vi "STM Read Message (TCP).vi"(6 "Options":T2={"Ignore Timeout Error"=TRUE, "timeout ms (1000)"=1000}, 8 "error in":errorcluster, 11 "Connection In":T4) -> (0 "error out":errorcluster, 1 "Name":T3, 2 "data string":string, 3 "Connection In":T4, 4 "Data Info":T1, 5 "Timed Out?":bool)   [LabVIEW 2015, in "J1939 Addon Shared.lvlib"]
doc: "This VI reads an incoming package of data from a host. This VI parses the package and extracts the data name and type as described in the meta data.\n\nFor the package to be parsed correctly, the meta data must be consistent in both the sender and the receiver. The data is packaged based on the existing meta data on the sender. \n\nUse the \"STM Read Meta Data\" and \"STM Write Meta Data\" VIs to ensure that both client and server have the same meta data.\n\nThe data is returned as a string. It is the responsibility of the user to cast it to the appropriate type."
uses:
  J1939 Addon Shared.lvlib
  stm_TCP Connection Info.ctl
  _SubVIs/stm_MetaDataElement.ctl
  stm_TCP Read Options.ctl
  stm_TCP Data Info.ctl
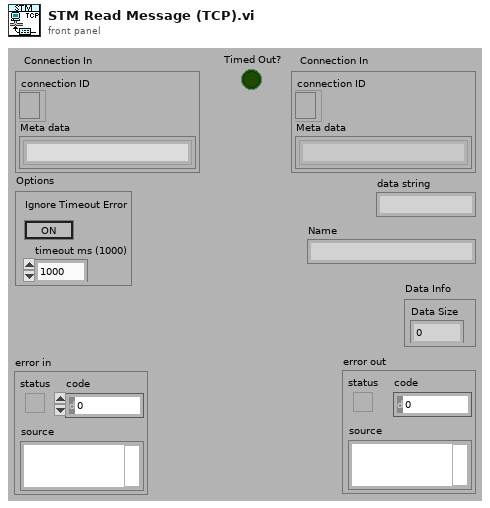
[diagram p1: front panel]
types:
  T1 = typedef "J1939 Addon Shared.lvlib/stm_TCP Data Info.ctl" = cluster{"Data Size":i32}
  T2 = typedef "J1939 Addon Shared.lvlib/stm_TCP Read Options.ctl" = cluster{"Ignore Timeout Error":bool, "timeout ms (1000)":i32}
  T3 = typedef "J1939 Addon Shared.lvlib/stm_MetaDataElement.ctl" = string
  T4 = typedef "J1939 Addon Shared.lvlib/stm_TCP Connection Info.ctl" = cluster{"connection ID":refnum<k5>, "Meta data":T3[]}
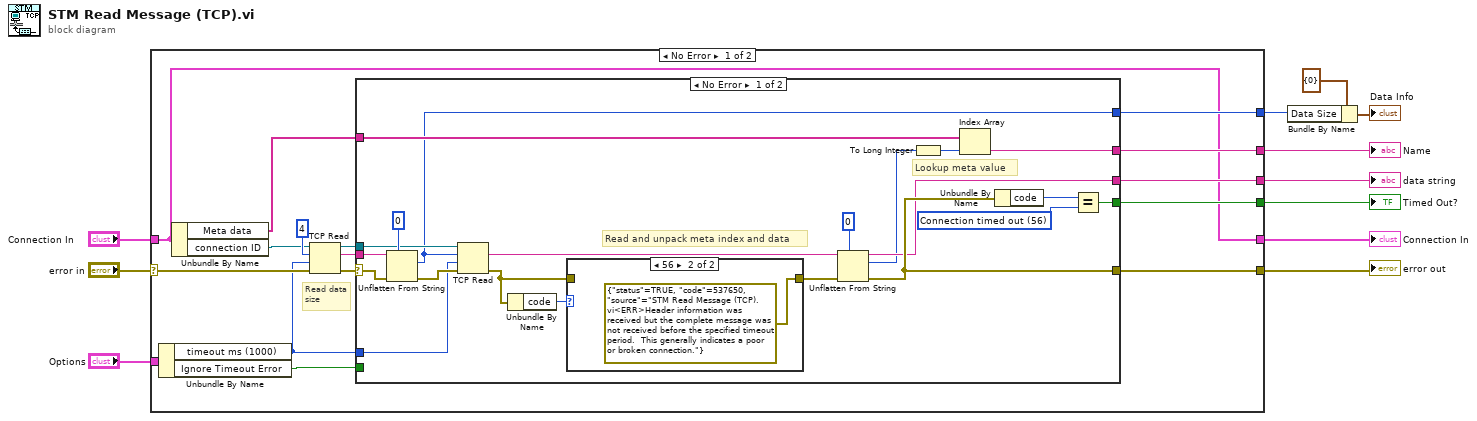
[diagram p0: block diagram]
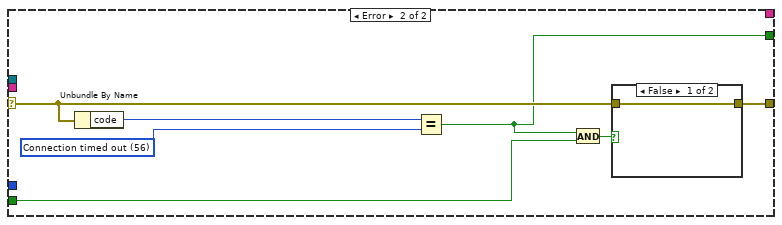
[diagram p3: hidden frame]
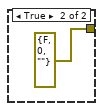
[diagram p4: hidden frame]
diagram:
  n1 = case shown="No Error" "error in" {
    selector: "error in" -> [w14 w60]
    tunnel: "Connection In" -> [w13 w61]
    tunnel: [w13 w61] -> w11
    tunnel: [w23 w60] -> w10
    tunnel: [w22 _] -> w9
    tunnel: [w21 _] -> w8
    tunnel: [w20 _] -> w7
    tunnel: [w19 _] -> w3
    tunnel: "Options" -> [w15 _]
    frame No Error {
      # "Read data size"
      n2 = Unbundle By Name(w15) -> ("timeout ms (1000)"=w12:i32, "Ignore Timeout Error"=w18:bool)
      n3 = Unbundle By Name(w13) -> ("Meta data"=w16:T3[], "connection ID"=w17:refnum<k5>)
      n4 = TCP Read(connection ID=w17, bytes to read=4, error in (no error)=w14, 9:w12) -> (connection ID out=w25:refnum<k5>, data out=w26:string, error out=w24:errorcluster)  [unwired: 1 out]
      n5 = case shown="No Error" w24 {
        selector: w24 -> [w41 w52]
        tunnel: w26 -> [w42 _]
        tunnel: w25 -> [w47 _]
        tunnel: w16 -> [w46 _]
        tunnel: [w40 w53] -> w23
        tunnel: w18 -> [_ w55]
        tunnel: [w43 w51] -> w22
        tunnel: [w39 _] -> w21
        tunnel: [w34 _] -> w20
        tunnel: [w38 _] -> w19
        tunnel: w12 -> [w28 _]
        frame No Error {
          w44 = 56 items=["No Error", "Argument Error", "Memory Full", "Out of Zone", "End of File", "File Already Open", "Generic File IO Error", "File Not Found", "File Permission Error", "Disk Full", "Duplicate Path", "Too Many Files Open", "Not Enabled", "Resource File Not Found", "Cannot Add Resource", "Resource Not Found", "Image Not Found", "Image Memory Error", "Pen Does Not Exist", "Config Bad Type", "Config Token Not Found", "Config Parse Error", "Config Memory Error", "Bad External Code Format", "Bad External Code Offset", "External Code Not Present", "Null Window", "Destroy Window Mixup", "Null Menu", "Print Aborted", "Bad Print Record", "Print Driver Error", "Windows Error During Print", "Memory Error During Print", "Print Dialog Error", "Generic Print Error", "Invalid Device Refnum", "Device Not Found", "Device Parameter Error", "Device Unit Error", "Can't Open Device", "Device Call Aborted", "Generic Error", "Cancelled By User", "Object ID Too Low", "Object ID Too High", "Object Not In Heap", "Unknown Heap", "Bad DefProc ID", "DefProc Not In Table", "Message Out Of Range", "Null Method", "Unknown Message", "Manager Call Not Supported", "Bad address", "Connection In progress", "Connection timed out", "Connection is already in progress", "Network attribute not supported", "Network error", "Address in use", "System out of memory", "Connection aborted", "Connection refused", "Connection is not connected", "Connection is already connected", "Connection closed", "Initialize error (interapplication manager)", "Bad occurrence", "Wait on unbound occurrence handler", "Occurrence queue overflow", "Bad path", "Semaphore not signaled", "Unrecognized type (interapplication manager)"] ("1st Error to Convert")
          # "Lookup meta value"
          # "Read and unpack meta index and data"
          n6 = Unflatten From String(type=0 ("bytes to read"), binary string=w42, error in (no error)=w41) -> (value=w38:i32, error out=w36:errorcluster)  [unwired: 1 in, 2 out]
          n7 = TCP Read(connection ID=w47, bytes to read=w38, error in (no error)=w36, 9:w28) -> (data out=w37:string, error out=w30:errorcluster)  [unwired: 2 out]
          n8 = Unbundle By Name(w30) -> ("code"=w29:i32)
          n9 = case shown="56" w29 {
            tunnel: w30 -> [w49 _]
            tunnel: [w49 errorcluster {"status"=TRUE, "code"=537650, "source"="STM Read Message (TCP).vi<ERR>Header information was received but the complete message was not received before the specified timeout period.  This generally indicates a poor or broken connection."} ("error out")] -> w31
            frame Default {
            }
            frame 56 {
            }
          }
          n10 = Unflatten From String(type=u16 0 ("bytes to read"), binary string=w37, error in (no error)=w31) -> (rest of the binary string=w34:string, value=w32:u16, error out=w40:errorcluster)  [unwired: 2 out]
          n11 = To Long Integer(number=w32) -> (32bit integer=w33:i32)
          n12 = Index Array(array=w46, index=w33) -> (element=w39:T3)
          n13 = Unbundle By Name(w40) -> ("code"=w45:i32)
          n14 = Equal?(x=w45, y=w44) -> (x = y?=w43:bool)
        }
        frame Error {
          w56 = 56 items=["No Error", "Argument Error", "Memory Full", "Out of Zone", "End of File", "File Already Open", "Generic File IO Error", "File Not Found", "File Permission Error", "Disk Full", "Duplicate Path", "Too Many Files Open", "Not Enabled", "Resource File Not Found", "Cannot Add Resource", "Resource Not Found", "Image Not Found", "Image Memory Error", "Pen Does Not Exist", "Config Bad Type", "Config Token Not Found", "Config Parse Error", "Config Memory Error", "Bad External Code Format", "Bad External Code Offset", "External Code Not Present", "Null Window", "Destroy Window Mixup", "Null Menu", "Print Aborted", "Bad Print Record", "Print Driver Error", "Windows Error During Print", "Memory Error During Print", "Print Dialog Error", "Generic Print Error", "Invalid Device Refnum", "Device Not Found", "Device Parameter Error", "Device Unit Error", "Can't Open Device", "Device Call Aborted", "Generic Error", "Cancelled By User", "Object ID Too Low", "Object ID Too High", "Object Not In Heap", "Unknown Heap", "Bad DefProc ID", "DefProc Not In Table", "Message Out Of Range", "Null Method", "Unknown Message", "Manager Call Not Supported", "Bad address", "Connection In progress", "Connection timed out", "Connection is already in progress", "Network attribute not supported", "Network error", "Address in use", "System out of memory", "Connection aborted", "Connection refused", "Connection is not connected", "Connection is already connected", "Connection closed", "Initialize error (interapplication manager)", "Bad occurrence", "Wait on unbound occurrence handler", "Occurrence queue overflow", "Bad path", "Semaphore not signaled", "Unrecognized type (interapplication manager)"] ("1st Error to Convert")
          n15 = Unbundle By Name(w52) -> ("code"=w57:i32)
          n16 = Equal?(x=w57, y=w56) -> (x = y?=w51:bool)
          n17 = And(x=w51, y=w55) -> (x .and. y?=w54:bool)
          n18 = case shown="False" w54 {
            tunnel: [w58 errorcluster {"status"=FALSE, "code"=0, "source"=""} ("error out")] -> w53
            tunnel: w52 -> [w58 _]
            frame False {
            }
            frame True {
            }
          }
        }
      }
    }
    frame Error {
    }
  }
  "error out" <- w10
  "Connection In" <- w11
  "Timed Out?" <- w9
  "data string" <- w7
  "Name" <- w8
  n19 = Bundle By Name(cluster=T1 {"Data Size"=0} ("Data Info"), "Data Size"=w3) -> (→"Data Info":T1)
